vi "getNyaNext.vi"(1 "saveNya?":bool, 2 "getNya?":bool) -> (0 "Nya":picture)   [LabVIEW 2014]
uses:
  <vilib>/Utility/miscctls.llb/LVBoundsTypeDef.ctl
  <vilib>/Utility/sysdir.llb/System Directory Type.ctl
  <vilib>/Platform/browser.llb/Open URL in Default Browser (string).vi
panel:
  out "reGetNya":bool
  out "fileNumber":i64
  out "numberOfTheNyas":i64
  in  "don'tWantNoMoreNya?":bool
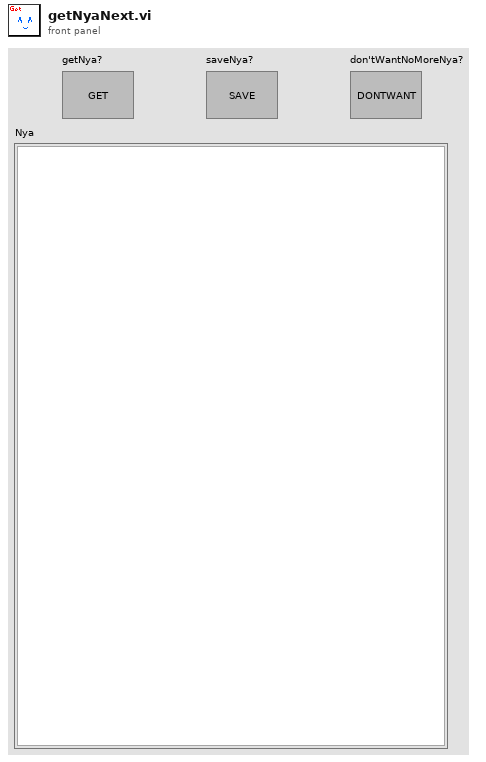
[diagram p1: front panel]
types:
  T1 = typedef "LVBoundsTypeDef.ctl" = cluster{"Width":u32, "Height":u32}
  T2 = typedef "imagedata.ctl" = cluster{"image type":i32, "image depth":i32, "image":u8[], "mask":u8[], "colors":u32[], "Rectangle":cluster{"left":i16, "top":i16, "right":i16, "bottom":i16}}
  T3 = typedef "System Directory Type.ctl" = i32
  T4 = enum16{"Native", "Native Command Line", "UNIX", "Macintosh", "DOS"}
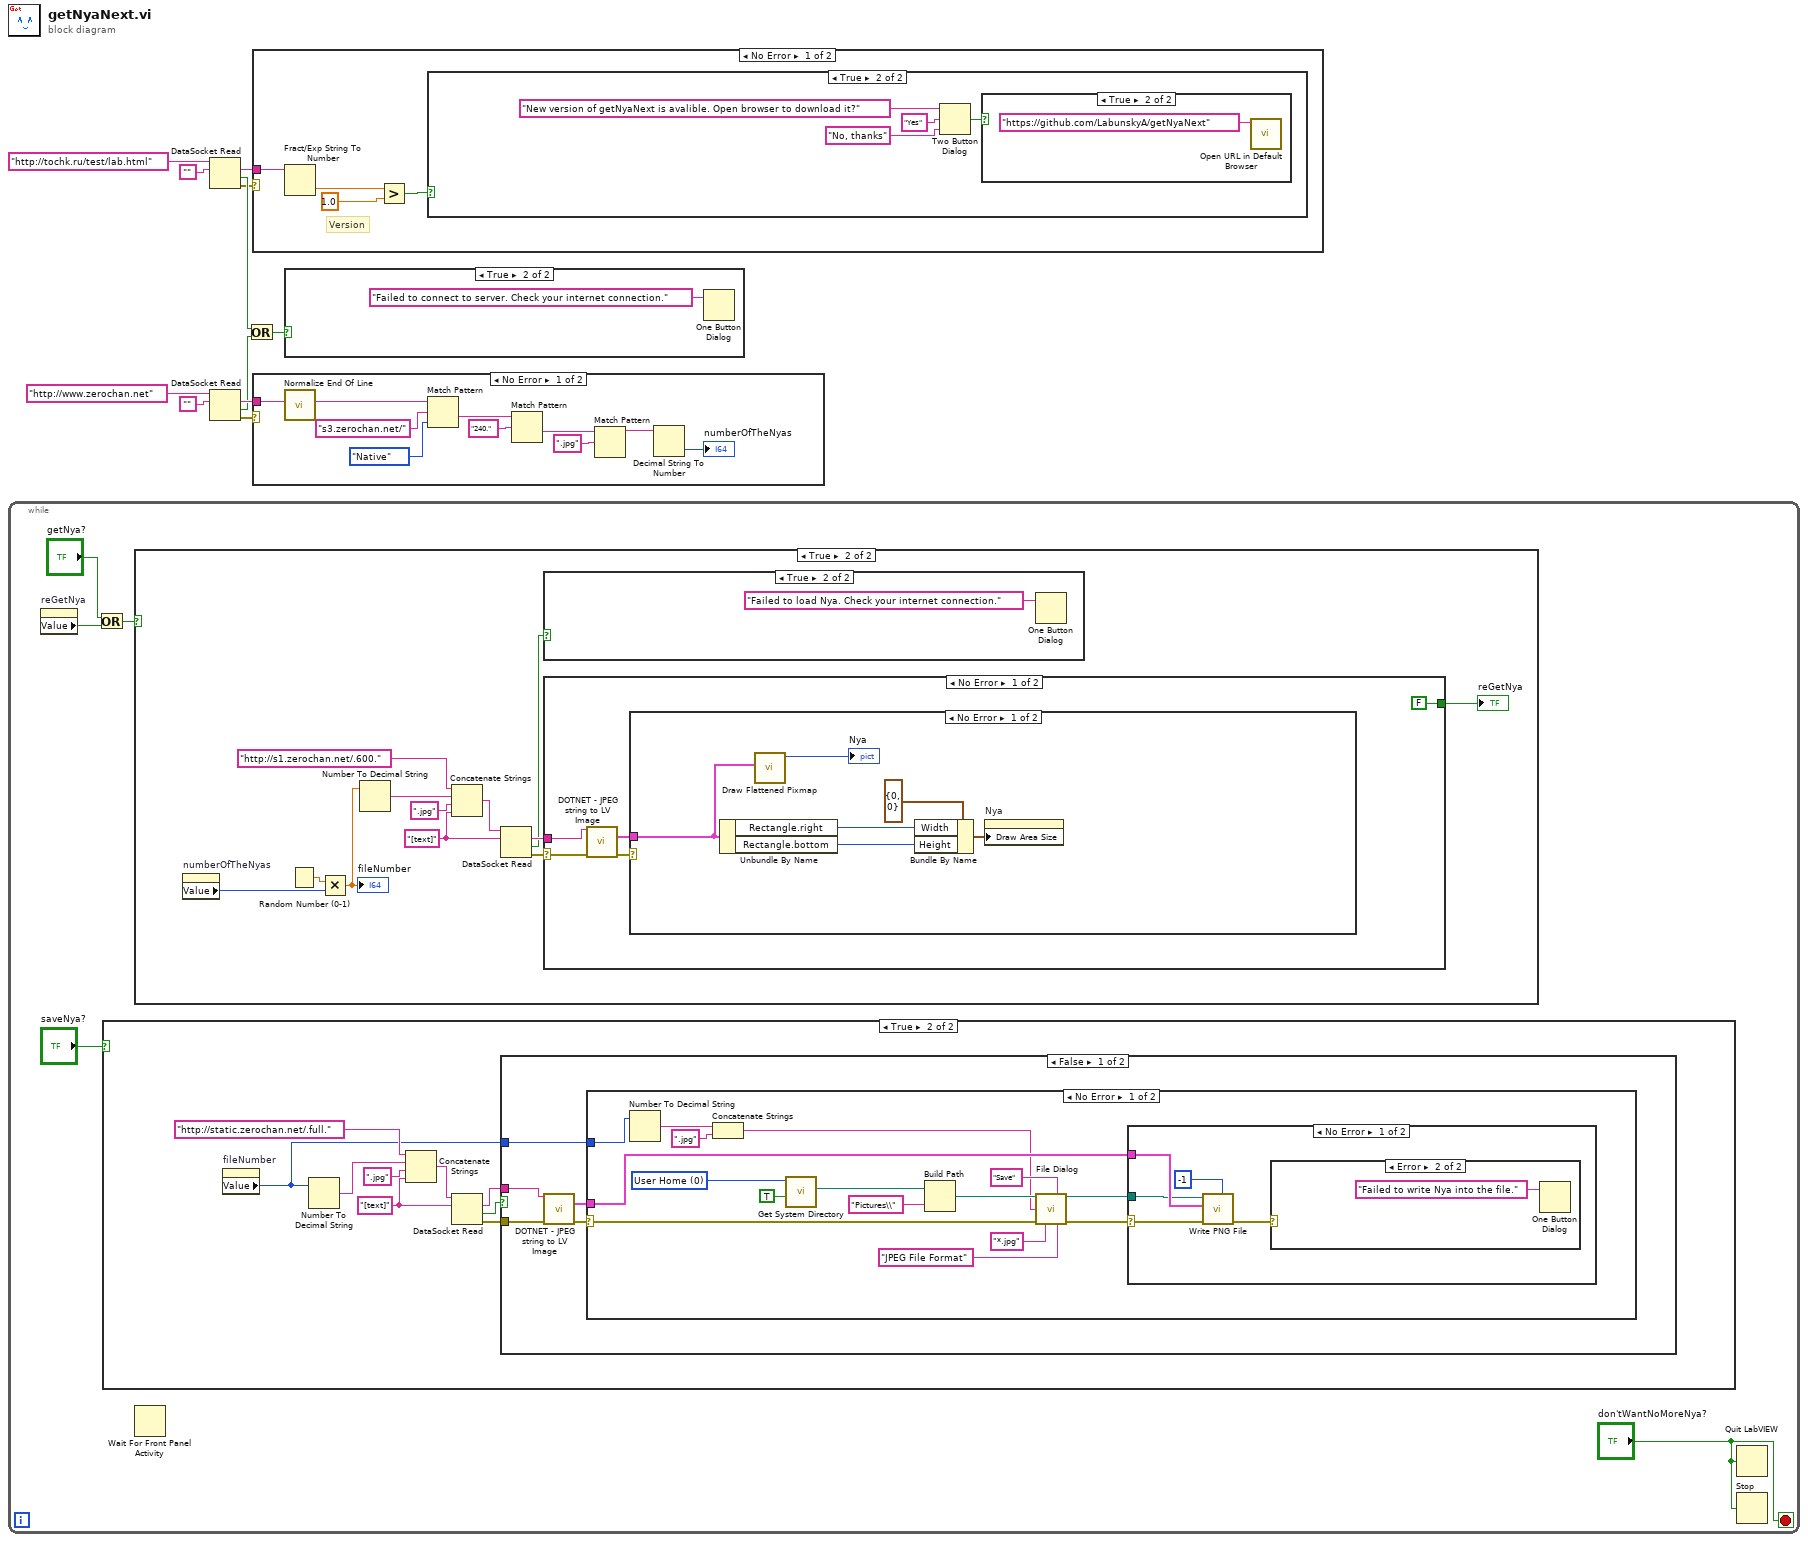
[diagram p0: block diagram]
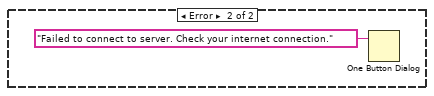
[diagram p5: hidden frame]
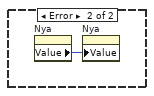
[diagram p9: hidden frame]
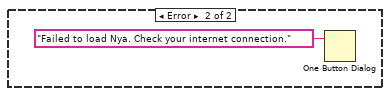
[diagram p10: hidden frame]
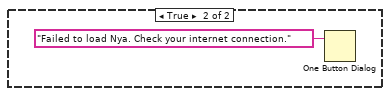
[diagram p11: hidden frame]
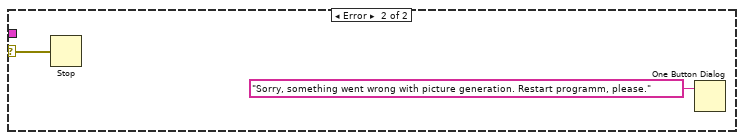
[diagram p14: hidden frame]
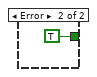
[diagram p15: hidden frame]
diagram:
  n1 = while {
    stop <- "don'tWantNoMoreNya?" stop-if-true
    n2 = property on="reGetNya" class="Bool (strict)"() -> ("Value"=w13:bool)  [unwired: 2 in, 2 out]
    n3 = Or(x="getNya?", y=w13) -> (x .or. y?=w14:bool)
    n4 = case shown="True" "saveNya?" {
      frame False {
      }
      frame True {
        w22 = "[text]"
        n5 = property on="fileNumber" class="DigNum (strict)"() -> ("Value"=w17:i64)  [unwired: 2 in, 2 out]
        n6 = Number To Decimal String(number=w17) -> (decimal integer string=w24:string)  [unwired: 1 in]
        n7 = Concatenate Strings("http://static.zerochan.net/.full.", w24, ".jpg", w22) -> (w23:string)
        n8 = DataSocket Read(10:w22, 11:w23) -> (0:w20:errorcluster, 1:w18:bool, 2:w21:string)  [unwired: 3 in, 4 out]
        n9 = case shown="False" w18 {
          tunnel: w21 -> [w30 _]
          tunnel: w20 -> [w29 _]
          tunnel: w17 -> [w26 _]
          frame False {
            n10 = call "DOTNET - JPEG string to LV Image.vi"("JPEG String"=w30, "error in"=w29) -> ("LV Image"=w28:T2, "error out"=w27:errorcluster)  [unwired: 12 in]
            n11 = case shown="No Error" w27 {
              selector: w27 -> [w43 _]
              tunnel: w28 -> [w46 _]
              tunnel: w26 -> [w31 _]
              frame No Error {
                w37 = T3 0 items=["User Home"=0, "User Desktop"=1, "User Documents"=2, "User Application Data"=3, "User Preferences"=4, "User Temporary"=5, "Public Documents"=6, "Public Application Data"=7, "Public Preferences"=8, "Public Cache"=13, "System Core Libraries"=9, "System Installed Libraries"=10, "Application Files"=11, "Boot Volume Root"=12] ("system directory type")
                n12 = Number To Decimal String(number=w31) -> (decimal integer string=w33:string)  [unwired: 1 in]
                n13 = Concatenate Strings(w33, ".jpg") -> (w32:string)
                n14 = call <vilib>:"Get System Directory.vi"("create directory if not found? (F)"=TRUE, "system directory type"=w37) -> ("system directory"=w38:path)  [unwired: 9 in]
                n15 = Build Path(base path=w38, name or relative path="Pictures\\") -> (appended path=w36:path)
                n16 = call "File Dialog"("start path"=w36, "button label"="Save", "default name"=w32, "error in"=w43, "pattern (all files)"="*.jpg", "pattern label"="JPEG File Format") -> ("selected path"=w45:path, "error out"=w44:errorcluster)  [unwired: 6 in, 2 out]
                n17 = case shown="No Error" w44 {
                  selector: w44 -> [w49 _]
                  tunnel: w46 -> [w51 _]
                  tunnel: w45 -> [w48 _]
                  frame No Error {
                    n18 = call <vilib>:"Write PNG File.vi"("compression (default)"=-1, "error in (no error)"=w49, "image data"=w51, "path to PNG file"=w48) -> ("error out"=w50:errorcluster)  [unwired: 6 in, 1 out]
                    n19 = case shown="Error" w50 {
                      frame No Error {
                      }
                      frame Error {
                        n20 = One Button Dialog(message="Failed to write Nya into the file.") -> ()  [unwired: 1 in, 1 out]
                      }
                    }
                  }
                  frame Error {
                    n21 = property on="Nya" class="Pict"() -> ("Value"=w53:picture)  [unwired: 2 in, 2 out]
                    n22 = property on="Nya" class="Pict"("Value"=w53) -> ()  [unwired: 2 in, 2 out]
                  }
                }
              }
              frame Error {
                n23 = One Button Dialog(message="Failed to load Nya. Check your internet connection.") -> ()  [unwired: 1 in, 1 out]
              }
            }
          }
          frame True {
            n24 = One Button Dialog(message="Failed to load Nya. Check your internet connection.") -> ()  [unwired: 1 in, 1 out]
          }
        }
      }
    }
    n25 = case shown="True" w14 {
      frame False {
      }
      frame True {
        w63 = "[text]"
        n26 = property on="numberOfTheNyas" class="DigNum (strict)"() -> ("Value"=w56:i64)  [unwired: 2 in, 2 out]
        n27 = Random Number (0-1)() -> (number: 0 to 1=w66:dbl)
        n28 = Multiply(x=w66, y=w56) -> (x*y=w59:dbl)
        "fileNumber" <- w59
        n29 = Number To Decimal String(number=w59) -> (decimal integer string=w65:string)  [unwired: 1 in]
        n30 = Concatenate Strings("http://s1.zerochan.net/.600.", w65, ".jpg", w63) -> (w67:string)
        n31 = DataSocket Read(10:w63, 11:w67) -> (0:w60:errorcluster, 1:w58:bool, 2:w62:string)  [unwired: 3 in, 4 out]
        n32 = case shown="True" w58 {
          frame False {
          }
          frame True {
            n33 = One Button Dialog(message="Failed to load Nya. Check your internet connection.") -> ()  [unwired: 1 in, 1 out]
          }
        }
        n34 = case shown="No Error" w60 {
          selector: w60 -> [w72 _]
          tunnel: w62 -> [w73 _]
          tunnel: [FALSE TRUE] -> w57
          frame No Error {
            n35 = call "DOTNET - JPEG string to LV Image.vi"("JPEG String"=w73, "error in"=w72) -> ("LV Image"=w70:T2, "error out"=w71:errorcluster)  [unwired: 12 in]
            n36 = case shown="No Error" w71 {
              selector: w71 -> [_ w81]
              tunnel: w70 -> [w74 _]
              frame No Error {
                n37 = Unbundle By Name(w74) -> ("Rectangle.right"=w78:i16, "Rectangle.bottom"=w79:i16)
                n38 = call <vilib>:"Draw Flattened Pixmap.vi"("image data"=w74) -> ("new picture"=→"Nya":picture)  [unwired: 8 in]
                n39 = Bundle By Name(cluster=T1 {"Width"=0, "Height"=0} ("Draw Area Size"), "Width"=w78, "Height"=w79) -> (w77:T1)
                n40 = property on="Nya" class="Pict"("Draw Area Size"=w77) -> ()  [unwired: 2 in, 2 out]
              }
              frame Error {
                n41 = Stop(stop? (T)=w81) -> ()
                n42 = One Button Dialog(message="Sorry, something went wrong with picture generation. Restart programm, please.") -> ()  [unwired: 1 in, 1 out]
              }
            }
          }
          frame Error {
          }
        }
        "reGetNya" <- w57
      }
    }
    n43 = Wait For Front Panel Activity() -> ()  [unwired: 3 in, 1 out]
    n44 = Quit LabVIEW(quit? (T)="don'tWantNoMoreNya?") -> ()
    n45 = Stop(stop? (T)="don'tWantNoMoreNya?") -> ()
  }
  n46 = DataSocket Read(10:"", 11:"http://tochk.ru/test/lab.html") -> (0:w2:errorcluster, 1:w4:bool, 2:w1:string)  [unwired: 3 in, 4 out]
  n47 = DataSocket Read(10:"", 11:"http://www.zerochan.net") -> (0:w9:errorcluster, 1:w3:bool, 2:w8:string)  [unwired: 3 in, 4 out]
  n48 = Or(x=w4, y=w3) -> (x .or. y?=w5:bool)
  n49 = case shown="No Error" w2 {
    tunnel: w1 -> [w86 _]
    frame No Error {
      # "Version"
      n50 = Fract/Exp String To Number(string=w86) -> (number=w84:dbl)  [unwired: 3 in, 1 out]
      n51 = Greater?(x=w84, y=1.0) -> (0:w83:bool)
      n52 = case shown="True" w83 {
        frame False {
        }
        frame True {
          n53 = Two Button Dialog(message="New version of getNyaNext is avalible. Open browser to download it?", 1:"No, thanks" ("F button name (\"Cancel\")"), 2:"Yes" ("T button name (\"OK\")")) -> (T button?=w87:bool)
          n54 = case shown="True" w87 {
            frame False {
            }
            frame True {
              n55 = call-poly <vilib>:"Open URL in Default Browser.vi"("URL"="https://github.com/LabunskyA/getNyaNext") -> ()  [unwired: 5 in, 2 out]
            }
          }
        }
      }
    }
    frame Error {
    }
  }
  n56 = case shown="No Error" w9 {
    tunnel: w8 -> [w92 _]
    frame No Error {
      n57 = call <vilib>:"Normalize End Of Line.vi"("string in"=w92) -> ("string out"=w101:string)  [unwired: 7 in]
      n58 = Match Pattern(string=w101, regular expression="s3.zerochan.net/", offset (0)=T4."Native" ("end of line (Native)")) -> (after substring=w98:string)  [unwired: 3 out]
      n59 = Match Pattern(string=w98, regular expression="240.") -> (after substring=w99:string)  [unwired: 1 in, 3 out]
      n60 = Match Pattern(string=w99, regular expression=".jpg") -> (before substring=w100:string)  [unwired: 1 in, 3 out]
      n61 = Decimal String To Number(string=w100) -> (number=→"numberOfTheNyas":i32)  [unwired: 2 in, 1 out]
    }
    frame Error {
      n62 = One Button Dialog(message="Failed to connect to server. Check your internet connection.") -> ()  [unwired: 1 in, 1 out]
    }
  }
  n63 = case shown="True" w5 {
    frame False {
    }
    frame True {
      n64 = One Button Dialog(message="Failed to connect to server. Check your internet connection.") -> ()  [unwired: 1 in, 1 out]
    }
  }
